vi "webcame bağlanma ve foto çekme.vi"() -> ()   [LabVIEW 2017]
uses:
  <vilib>/userdefined/High Color/IMAQdx.ctl
  <vilib>/vision/driver/NI_Vision_Acquisition_Software.lvlib
panel:
  in  "camera stop":bool
  out "Image":T1(plugin-control)
  in  "Photo":bool
  out "error out 3":errorcluster
  out "error out 2":errorcluster
  out "error out":errorcluster
  in  "selection camera":T2
  in  "Search Rect (entire image)":T3 {"Rotation" format="%.2f"; "Left" scale=0.0..1024.0; "Right" scale=0.0..1024.0}
  out "Number of Objects":i32
  out "error out 4":errorcluster
  in  "Settings":T4={"Objects"=0, "Threshold"=128, "Reject Border"=FALSE, "Fill Holes"=FALSE, "Min Object Size"=FALSE, "Min Size"=3, "Max Object Size"=FALSE, "Max Size"=100, "Show Search Area"=FALSE, "Show Center"=TRUE, "Show Bounding Box"=TRUE} {"Objects" items=["Bright Objects", "Dark Objects"]; "Threshold" min=1 max=999999999 step=1; "Max Size" min=1 max=999999999 step=1; "Min Size" min=1 max=999999999 step=1}
  in  "File Path":path
  out "Uygulanan İşlem":T1(plugin-control)
  in  "Image Type":T5 items=["Grayscale (U8)", "Grayscale (I16)", "Grayscale (SGL)", "Complex (CSG)", "RGB (U32)", "HSL (U32)", "RGB (U64)", "Grayscale (U16)"]
  in  "operations stop":bool
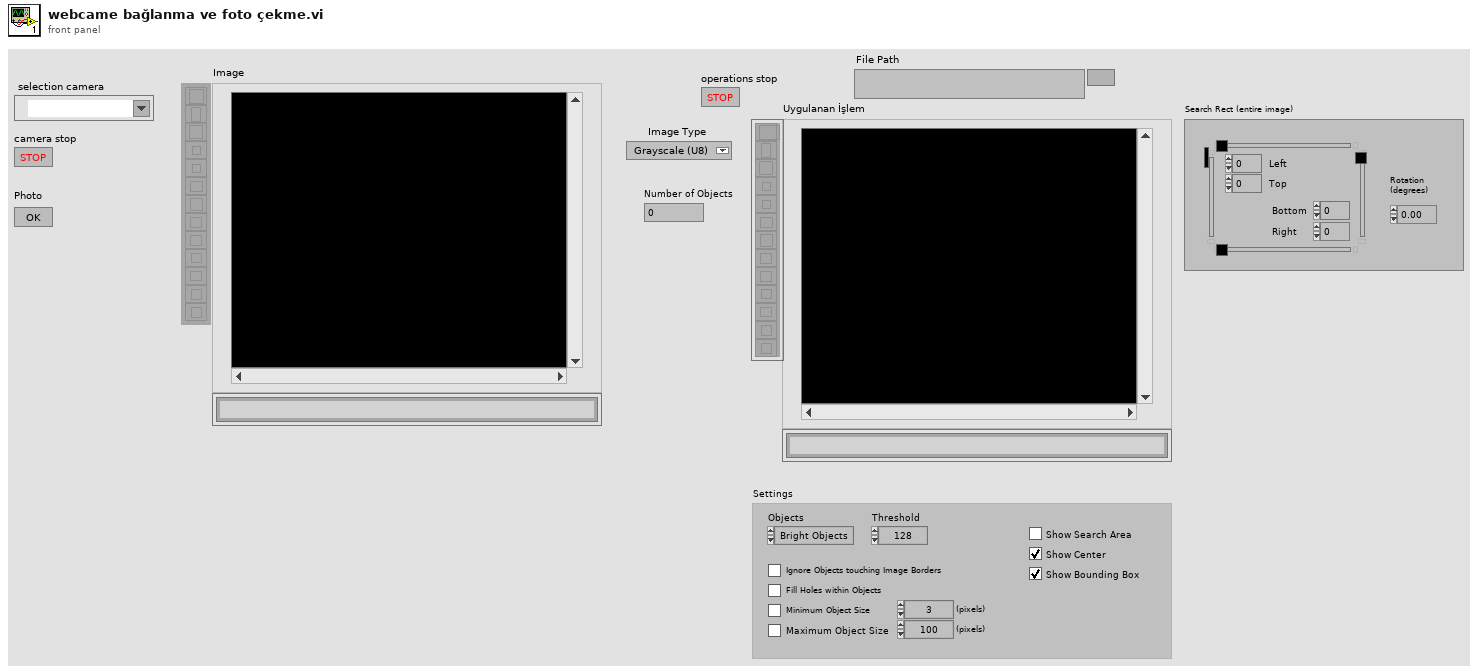
[diagram p1: front panel]
types:
  T1 = typedef "IMAQ Image.ctl" = refnum<image>
  T2 = typedef "IMAQdx.ctl" = refnum<k21>
  T3 = typedef "IMAQ Rectangle" = cluster{"Left":i32, "Top":i32, "Right":i32, "Bottom":i32, "Rotation":dbl}
  T4 = cluster{"Objects":u16, "Threshold":i32, "Reject Border":bool, "Fill Holes":bool, "Min Object Size":bool, "Min Size":i32, "Max Object Size":bool, "Max Size":i32, "Show Search Area":bool, "Show Center":bool, "Show Bounding Box":bool}
  T5 = typedef "Image Type" = u32
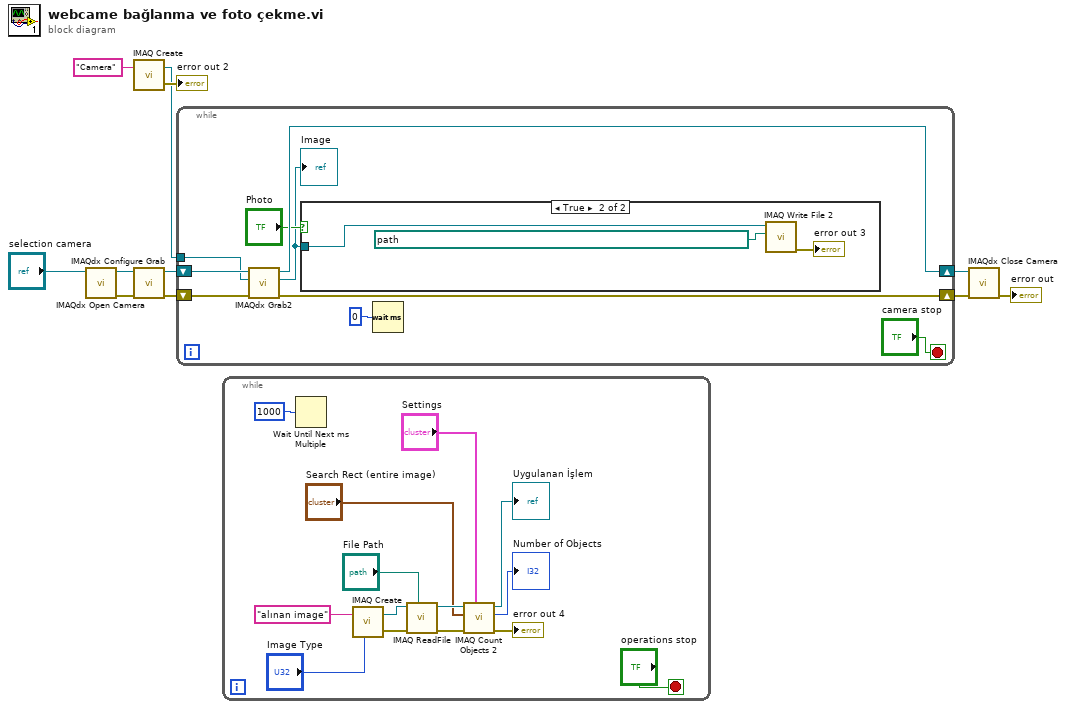
[diagram p0: block diagram]
diagram:
  n1 = call <vilib>:"IMAQdx Open Camera.vi"("Session In"="selection camera") -> ("error out"=w9:errorcluster, "Session Out"=w10:T2)  [unwired: 9 in]
  n2 = call "IMAQ Create"("Image Name"="Camera") -> ("New Image"=w4:T1, "error out"=→"error out 2":errorcluster)  [unwired: 4 in]
  n3 = call <vilib>:"IMAQdx Configure Grab.vi"("error in"=w9, "Session In"=w10) -> ("error out"=w7:errorcluster, "Session Out"=w8:T2)  [unwired: 8 in]
  n4 = while {
    tunnel: w4 -> [w16]
    shift-right: [w17] -> w3
    shift-left: w8 -> [w20]
    shift-right: [w18] -> w2
    shift-left: w7 -> [w19]
    stop <- "camera stop" stop-if-true
    n5 = call <vilib>:"IMAQdx Grab2.vi"("error in"=w19, "Image In"=w16, "Session In"=w20) -> ("error out"=w18:errorcluster, "Image Out"=w12:T1, "Session Out"=w17:T2)  [unwired: 5 in, 1 out]
    "Image" <- w12
    n6 = case shown="True" "Photo" {
      tunnel: w12 -> [_ w23]
      frame False {
      }
      frame True {
        n7 = call-poly "IMAQ Write File 2"("File Path"=path "D:/Yedek Masaüstü/Computer Aided Engineering 2/Proje/image.jpg", "Image"=w23) -> ("error out"=→"error out 3":errorcluster)  [unwired: 8 in, 1 out]
      }
    }
    n8 = Wait (ms)(milliseconds to wait=u32 0) -> ()  [unwired: 1 out]
  }
  n9 = while {
    stop <- "operations stop" stop-if-true
    n10 = Wait Until Next ms Multiple(millisecond multiple=u32 1000) -> ()  [unwired: 1 out]
    n11 = call "IMAQ Create"("Image Name"="alınan image", "Image Type"="Image Type") -> ("New Image"=w34:T1, "error out"=w28:errorcluster)  [unwired: 3 in]
    n12 = call "IMAQ ReadFile"("File Path"="File Path", "error in (no error)"=w28, "Image"=w34) -> ("error out"=w27:errorcluster, "Image Out"=w33:T1)  [unwired: 4 in, 3 out]
    n13 = call "IMAQ Count Objects 2"("Settings"="Settings", "error in (no error)"=w27, "Search Rect (entire image)"="Search Rect (entire image)", "Image"=w33) -> ("error out"=→"error out 4":errorcluster, "Number of Objects"=→"Number of Objects":i32, "Image Out"=→"Uygulanan İşlem":T1)  [unwired: 3 in, 2 out]
  }
  n14 = call <vilib>:"IMAQdx Close Camera.vi"("error in"=w2, "Session In"=w3) -> ("error out"=→"error out":errorcluster)  [unwired: 9 in]
